vi "ReImToMagPhase.vi"(10 "Im":dbl[](array[numeric]), 11 "Re":dbl[](array[numeric])) -> (2 "Phase":dbl[](array[numeric]), 3 "Mag":dbl[](array[numeric]))   [LabVIEW 2021]
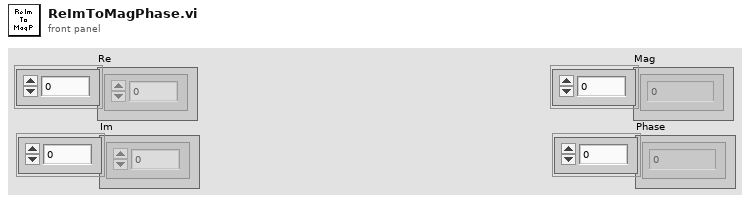
[diagram p1: front panel]
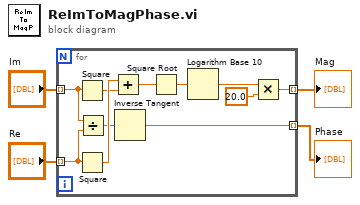
[diagram p0: block diagram]
diagram:
  n1 = for {
    tunnel: "Re" -> [w10] mode=indexing
    tunnel: "Im" -> [w11] mode=indexing
    tunnel: [w5] -> w2 mode=indexing
    tunnel: [w9] -> w1 mode=indexing
    n2 = Square(x=w11) -> (x^2=w12:dbl)
    n3 = Square(x=w10) -> (x^2=w15:dbl)
    n4 = Divide(x=w11, y=w10) -> (x/y=w13:dbl)
    n5 = Add(x=w15, y=w12) -> (x+y=w14:dbl)
    n6 = Inverse Tangent(1:w13) -> (0:w9:dbl)
    n7 = Square Root(x=w14) -> (sqrt(x)=w8:dbl)
    n8 = Logarithm Base 10(1:w8) -> (0:w7:dbl)
    n9 = Multiply(x=w7, y=20.0) -> (x*y=w5:dbl)
  }
  "Mag" <- w2
  "Phase" <- w1
